vi "Acquisition & Save MC.vi"() -> ()   [LabVIEW 2012]
doc: "© Copyright M. Ferrari 2004"
uses:
  <vilib>/Utility/file.llb/Write To Spreadsheet File (DBL).vi
panel:
  out "String":string="visible"
  out "Table":string[][](table)
  in  "Start":bool caption="ok"
  in  "stop":bool caption="ok"
  in  "append":bool
  in  "save":bool
  in  "Tc (sec)":sgl=0.3 format="%.2f"
  in  "n° punti":i32=10
  out "msg":string="Misura in corso"
  out "tab":string[][](table)
  # "ACQUIRE & SAVE"
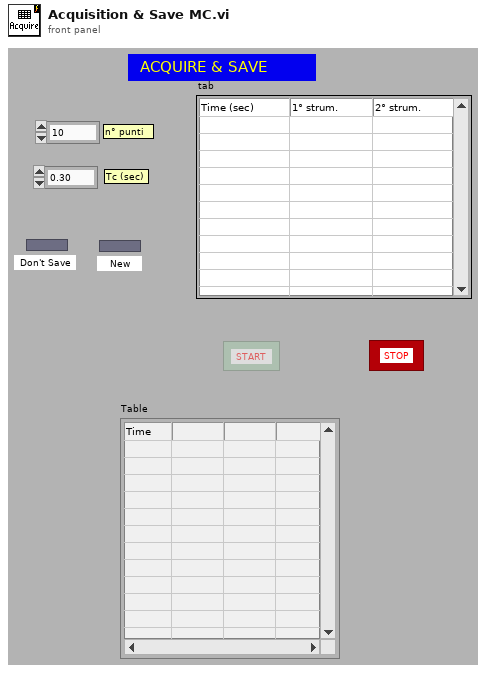
[diagram p1: front panel]
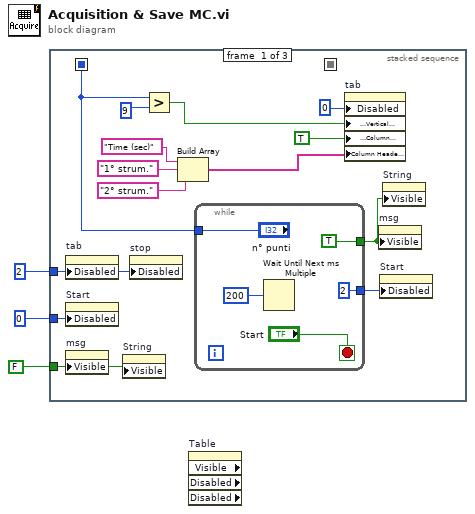
[diagram p0: block diagram]
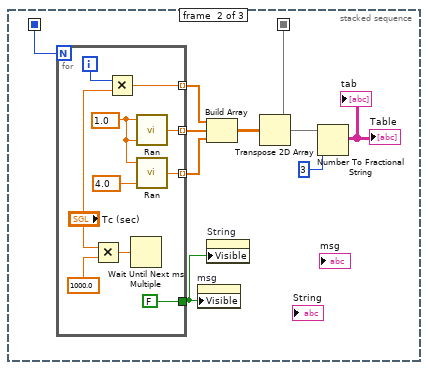
[diagram p2: hidden frame]
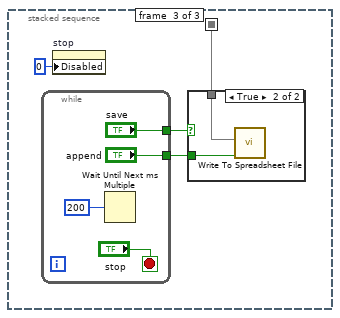
[diagram p3: hidden frame]
diagram:
  n1 = stacked-sequence {
    seq-local: [_ w26 _] -> [_ _ w43]
    seq-local: [w12 _ _] -> [_ w25 _]
    tunnel: u8 2 ("Disabled") -> [w6 _ _]
    tunnel: FALSE ("Visible") -> [w5 _ _]
    tunnel: u8 0 ("Disabled") -> [w9 _ _]
    frame #0 {
      n2 = property on="tab" class="Tbl (strict)"("Disabled"=w6) -> ()  [unwired: 2 in, 2 out]
      n3 = property on="Start" class="Bool"("Disabled"=w9) -> ()  [unwired: 2 in, 2 out]
      n4 = property on="msg" class="Str"("Visible"=w5) -> ()  [unwired: 2 in, 2 out]
      n5 = property on="String" class="Str"("Visible"=w5) -> ()  [unwired: 2 in, 2 out]
      n6 = property on="stop" class="Bool"("Disabled"=w6) -> ()  [unwired: 2 in, 2 out]
      n7 = Build Array("Time (sec)", "1° strum.", "2° strum.") -> (w8:string[])
      n8 = while {
        tunnel: [TRUE ("Visible")] -> w7
        tunnel: ["n° punti"] -> w12
        tunnel: [u8 2 ("Disabled")] -> w4
        stop <- "Start" stop-if-true
        n9 = Wait Until Next ms Multiple(millisecond multiple=u32 200) -> ()  [unwired: 1 out]
      }
      n10 = Greater?(x=w12, y=9) -> (0:w10:bool)
      n11 = property on="tab" class="Tbl (strict)"("Disabled"=u8 0, "Visible Items:Vertical Scrollbar Visible"=w10, "Visible Items:Column Headers Visible"=TRUE ("Column Headers Visible"), "Column Header Strings[]"=w8) -> ()  [unwired: 2 in, 2 out]
      n12 = property on="msg" class="Str"("Visible"=w7) -> ()  [unwired: 2 in, 2 out]
      n13 = property on="Start" class="Bool"("Disabled"=w4) -> ()  [unwired: 2 in, 2 out]
      n14 = property on="String" class="Str"("Visible"=w7) -> ()  [unwired: 2 in, 2 out]
    }
    frame #1 {
      n15 = for {
        N: w25 -> [_]
        tunnel: [w39] -> w29 mode=indexing
        tunnel: [w38] -> w31 mode=indexing
        tunnel: [FALSE ("Visible")] -> w23
        tunnel: [w32] -> w28 mode=indexing
        i -> [w34]
        w41 = 1.0 ("mul fatt")
        n16 = Multiply(x="Tc (sec)", y=sgl 1000.0) -> (x*y=w36:sgl)
        n17 = Multiply(x=w34, y="Tc (sec)") -> (x*y=w32:sgl)
        n18 = Wait Until Next ms Multiple(millisecond multiple=w36) -> ()  [unwired: 1 out]
        n19 = call "Ran.vi"("offset"=w41, "mul fatt"=w41) -> ("out num"=w39:dbl)  [unwired: 3 in]
        n20 = call "Ran.vi"("offset"=4.0, "mul fatt"=w41) -> ("out num"=w38:dbl)  [unwired: 3 in]
      }
      n21 = property on="msg" class="Str"("Visible"=w23) -> ()  [unwired: 2 in, 2 out]
      n22 = Build Array(w28, w29, w31) -> (w27:dbl[][])
      n23 = property on="String" class="Str"("Visible"=w23) -> ()  [unwired: 2 in, 2 out]
      n24 = Transpose 2D Array(2D array=w27) -> (transposed array=w26:dbl[][])
      n25 = Number To Fractional String(number=w26, precision (6)=3) -> (F-format string=→"tab" →"Table":string[][])  [unwired: 2 in]
    }
    frame #2 {
      n26 = while {
        tunnel: ["save"] -> w45
        tunnel: ["append"] -> w44
        stop <- "stop" stop-if-true
        n27 = Wait Until Next ms Multiple(millisecond multiple=u32 200) -> ()  [unwired: 1 out]
      }
      n28 = property on="stop" class="Bool"("Disabled"=u8 0) -> ()  [unwired: 2 in, 2 out]
      n29 = case shown="True" w45 {
        tunnel: w44 -> [_ w47]
        tunnel: w43 -> [_ w46]
        frame False {
        }
        frame True {
          n30 = call-poly <vilib>:"Write To Spreadsheet File.vi"("append to file? (new file:F)"=w47, "2D data"=w46) -> ()  [unwired: 6 in, 1 out]
        }
      }
    }
  }
  n31 = property on="Table" class="Tbl (strict)" props=["Visible", "Disabled", "Disabled"]() -> ()  [unwired: 2 in, 5 out]
